vi "gripper2.vi"() -> ()   [LabVIEW 2017]
uses:
  Program Files (x86)/National Instruments/LabVIEW 2017/examples/Instrument IO/Serial/support/Serial - Settings.ctl
  <vilib>/Instr/_visa.llb/VISA Configure Serial Port (Instr).vi
  Global 1.vi
panel:
  out "입력":string="*IDN?\n"
  in  "정지":bool
  out "Response":string
  out "bytes read":u32
  out "check":bool
  in  "Serial Settings":T1={"baud rate"=9600, "data bits"=8, "parity"=enum."None", "stop bits"=10, "flow control"=0} {"flow control" items=["None"=0, "XON/XOFF"=1, "RTS/CTS"=2, "DTR/DSR"=4]; "stop bits" items=["1.0"=10, "1.5"=15, "2.0"=20]; "data bits" min=5 max=8 step=1; "baud rate" items=["75"=75, "110"=110, "134"=134, "150"=150, "300"=300, "600"=600, "1200"=1200, "1800"=1800, "2400"=2400, "4800"=4800, "7200"=7200, "9600"=9600, "14400"=14400, "19200"=19200, "28800"=28800, "38400"=38400, "56000"=56000, "57600"=57600, "115200"=115200, "128000"=128000, "230400"=230400]}
  in  "delay before read (ms)":u32=500
  in  "VISA resource name":refnum<visa-resource-name>="COM1"
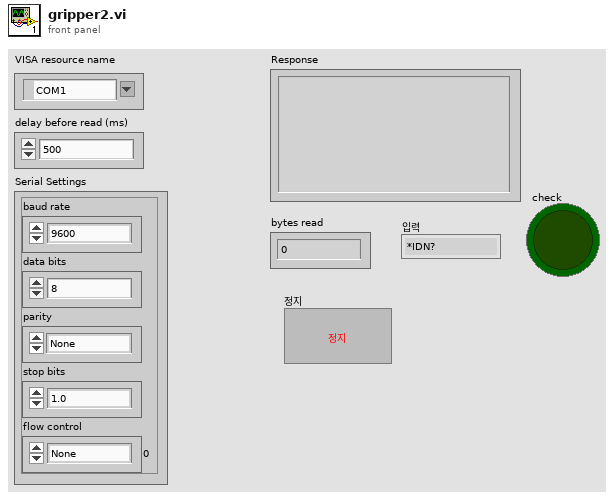
[diagram p1: front panel]
types:
  T1 = typedef "Serial - Settings.ctl" = cluster{"baud rate":u32, "data bits":u16, "parity":enum16{"None", "Odd", "Even", "Mark", "Space"}, "stop bits":u16, "flow control":u16}
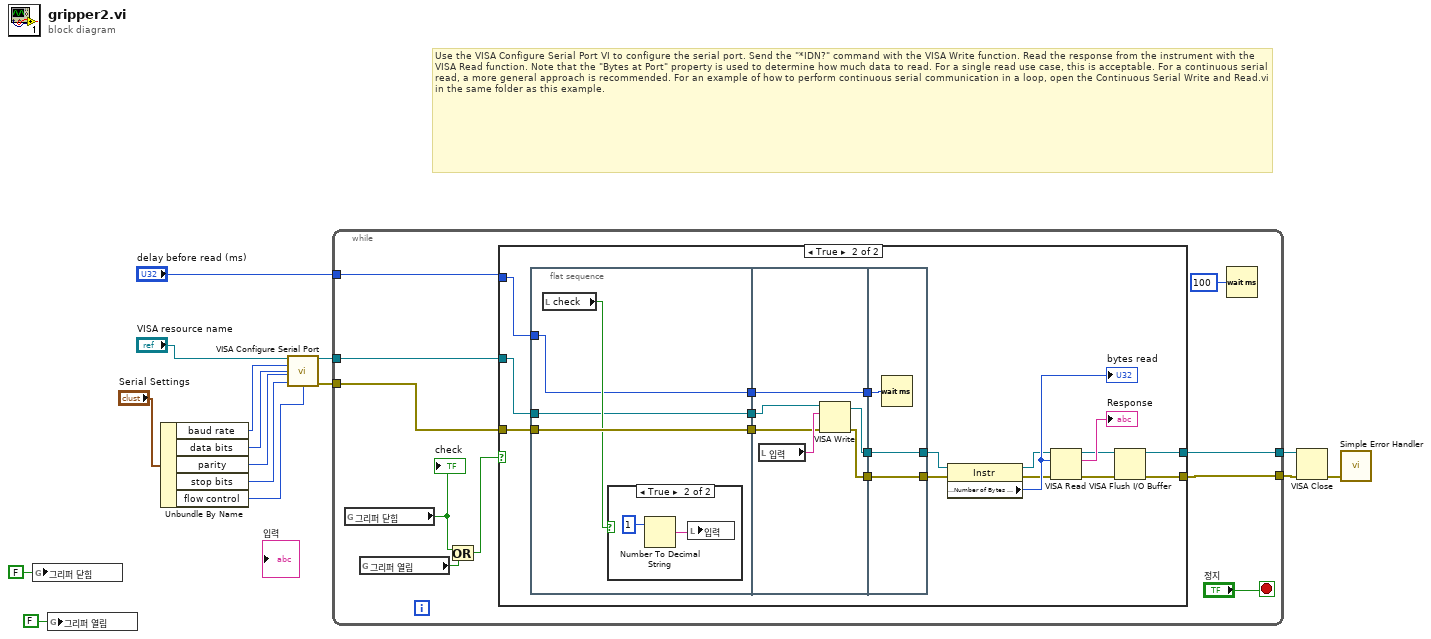
[diagram p0: block diagram]
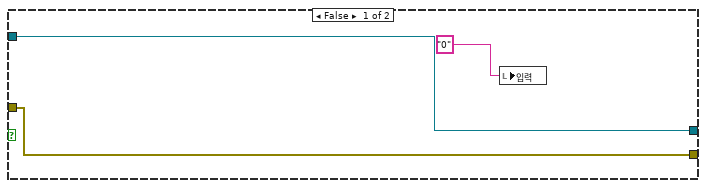
[diagram p2: hidden frame]
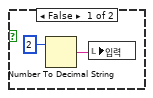
[diagram p3: hidden frame]
diagram:
  # "Use the VISA Configure Serial Port VI to configure the serial port. Send the \"*IDN?\" command with the VISA Write function. Read the response from the instrument with the VISA Read function. Note that the \"Bytes at Port\" property is used to determine how much data to read. For a single read use case, this is acceptable. For a continuous serial read, a more general approach is recommended. For an example of how to perform continuous serial communication in a loop, open the Continuous Serial Write and Read.vi in the same folder as this example."
  n1 = global write "Global 1.vi" "그리퍼 닫힘"(FALSE ("그리퍼 닫힘")) -> ()
  n2 = global write "Global 1.vi" "그리퍼 열림"(FALSE ("그리퍼 열림")) -> ()
  n3 = Unbundle By Name("Serial Settings") -> ("baud rate"=w12:u32, "data bits"=w11:u16, "parity"=w10:enum16{"None", "Odd", "Even", "Mark", "Space"}, "stop bits"=w9:u16, "flow control"=w8:u16)
  n4 = call-poly "VISA Configure Serial Port"("VISA resource name"="VISA resource name", "baud rate (9600)"=w12, "data bits (8)"=w11, "parity (0:none)"=w10, "stop bits (10: 1 bit)"=w9, "flow control (0:none)"=w8) -> ("VISA resource name out"=w7:refnum<visa-resource-name>, "error out"=w6:errorcluster)  [unwired: 3 in, 5 out]
  n5 = while {
    tunnel: "delay before read (ms)" -> [w22]
    tunnel: w7 -> [w20]
    tunnel: w6 -> [w21]
    tunnel: [w19] -> w5
    tunnel: [w18] -> w4
    stop <- "정지" stop-if-true
    n6 = global read "Global 1.vi" "그리퍼 닫힘"() -> (w16:bool)
    "check" <- w16
    n7 = global read "Global 1.vi" "그리퍼 열림"() -> (w17:bool)
    n8 = Or(x=w16, y=w17) -> (x .or. y?=w23:bool)
    n9 = case shown="True" w23 {
      tunnel: w22 -> [_ w37]
      tunnel: [w27 w30] -> w19
      tunnel: w21 -> [w27 w39]
      tunnel: w20 -> [w26 w33]
      tunnel: [w26 w29] -> w18
      frame False {
        n10 = local write "입력"("0") -> ()
      }
      frame True {
        n11 = flat-sequence {
          tunnel: w39 -> [w51]
          tunnel: [w51] -> w38
          tunnel: w37 -> [w49]
          tunnel: [w49] -> w35
          tunnel: [w48] -> w34
          tunnel: w33 -> [w48]
          tunnel: [w59] -> w41
          tunnel: [w58] -> w40
          tunnel: w38 -> [w60]
          tunnel: [w57] -> w36
          tunnel: w35 -> [w57]
          tunnel: w34 -> [w56]
          tunnel: [w64] -> w42
          tunnel: [w63] -> w43
          tunnel: w41 -> [w64]
          tunnel: w40 -> [w63]
          tunnel: w36 -> [w62]
          frame #0 {
            n12 = local read "check"() -> (w50:bool)
            n13 = case shown="True" w50 {
              frame False {
                n14 = Number To Decimal String(number=2 ("숫자")) -> (decimal integer string=w53:string)  [unwired: 1 in]
                n15 = local write "입력"(w53) -> ()
              }
              frame True {
                n16 = Number To Decimal String(number=1 ("숫자")) -> (decimal integer string=w55:string)  [unwired: 1 in]
                n17 = local write "입력"(w55) -> ()
              }
            }
          }
          frame #1 {
            n18 = local read "입력"() -> (w61:string)
            n19 = VISA Write(VISA resource name=w56, write buffer=w61, error in (no error)=w60) -> (VISA resource name out=w58:refnum<visa-resource-name>, error out=w59:errorcluster)  [unwired: 1 out]
          }
          frame #2 {
            n20 = Wait (ms)(milliseconds to wait=w62) -> ()  [unwired: 1 out]
          }
        }
        n21 = property class="Instr"(reference=w43, error in=w42) -> (reference out=w44:refnum<visa-resource-name>, error out=w45:errorcluster, "Serial Settings:Number of Bytes at Serial Port"=w47:u32)
        "bytes read" <- w47
        n22 = VISA Read(VISA resource name=w44, byte count=w47, error in (no error)=w45) -> (VISA resource name out=w32:refnum<visa-resource-name>, read buffer=→"Response":string, error out=w31:errorcluster)  [unwired: 1 out]
        n23 = VISA Flush I/O Buffer(VISA resource name=w32, error in (no error)=w31) -> (VISA resource name out=w29:refnum<visa-resource-name>, error out=w30:errorcluster)  [unwired: 1 in]
      }
    }
    n24 = Wait (ms)(milliseconds to wait=u32 100 ("대기 시간 (ms)")) -> ()  [unwired: 1 out]
  }
  n25 = VISA Close(VISA resource name=w4, error in (no error)=w5) -> (error out=w3:errorcluster)
  n26 = call <vilib>:"Simple Error Handler.vi"("error in (no error)"=w3) -> ()  [unwired: 1 in, 8 out]
